vi "MCL Get All Handles.vi"(10 "size":i32, 11 "handles":i32) -> (2 "function return":i32, 3 "handles out":i32)   [LabVIEW 2017, in "Madlib.lvlib"]
doc: "MADLIB_API int MCL_GetAllHandles(int *handles, int size);"
uses:
  Madlib.lvlib
  Madlib.dll
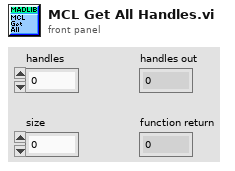
[diagram p1: front panel]
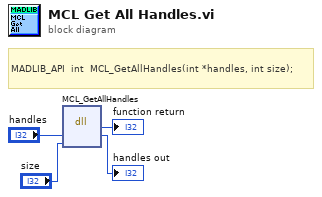
[diagram p0: block diagram]
diagram:
  # "MADLIB_API  int\t\tMCL_GetAllHandles(int *handles, int size);"
  n1 = dll-call lib="C:/Users/francesco/dev/pump-probe/Piezo/lvlib/Madlib.*" fn="MCL_GetAllHandles"("handles"="handles", "size"="size") -> (→"function return":i32, "handles"=→"handles out":i32)  [unwired: 4 in, 2 out]
